vi "Result.Merge Fault Code, Digit Fields, Use Highest Digit per Field.vi"(10 "Code2":i32 format="%010d", 11 "Code1":i32 format="%010d") -> (3 "Code Out":i32 format="%010d")   [LabVIEW 2019]
panel:
  out "Output":string
  out "Code2":string
  out "Code1":string
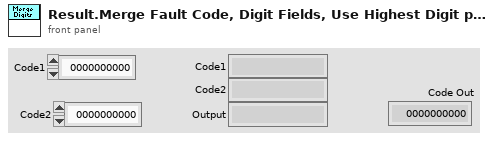
[diagram p1: front panel]
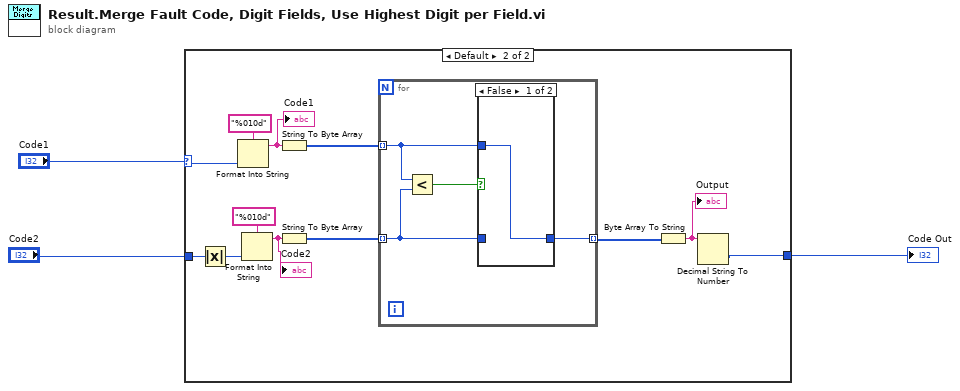
[diagram p0: block diagram]
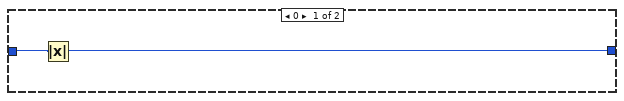
[diagram p2: hidden frame]
diagram:
  n1 = case shown="Default" "Code1" {
    selector: "Code1" -> [_ w13]
    tunnel: "Code2" -> [w5 w17]
    tunnel: [w4 w12] -> w1
    frame 0 {
      n2 = Absolute Value(x=w5) -> (abs(x)=w4:i32)
    }
    frame Default {
      n3 = Absolute Value(x=w17) -> (abs(x)=w14:i32)
      n4 = Format Into String(format string="%010d", w13) -> (resulting string=w11:string)  [unwired: 2 in, 1 out]
      "Code1" <- w11
      n5 = Format Into String(format string="%010d", w14) -> (resulting string=w10:string)  [unwired: 2 in, 1 out]
      "Code2" <- w10
      n6 = String To Byte Array(string=w11) -> (unsigned byte array=w8:u8[])
      n7 = String To Byte Array(string=w10) -> (unsigned byte array=w7:u8[])
      n8 = for {
        tunnel: w8 -> [w20] mode=indexing
        tunnel: w7 -> [w19] mode=indexing
        tunnel: [w21] -> w6 mode=indexing
        n9 = Less?(x=w20, y=w19) -> (x < y?=w18:bool)
        n10 = case shown="False" w18 {
          tunnel: w20 -> [w22 _]
          tunnel: w19 -> [_ w23]
          tunnel: [w22 w23] -> w21
          frame False {
          }
          frame True {
          }
        }
      }
      n11 = Byte Array To String(unsigned byte array=w6) -> (string=w9:string)
      "Output" <- w9
      n12 = Decimal String To Number(string=w9) -> (number=w12:i32)  [unwired: 2 in, 1 out]
    }
  }
  "Code Out" <- w1
